vi "PH_SHS_Analysis.PC Global On.vi"(0 "i ref in":refnum<vi>, 2 "Global On?":bool, 5 "error in (no error)":errorcluster) -> (14 "i ref out":refnum<vi>, 19 "error out":errorcluster)   [LabVIEW 2014, in "PH_SHS_Analysis.lvlib"]
doc: "This is the Proc Case \"Remote Control\"."
uses:
  PH_SHS_Analysis.lvlib
  PH_Common/PH_Common.lvlib
  CSCore/BaseProcess/BaseProcess.lvlib
  PH_Img_BaseClass/PH_Img_BaseClass.lvlib
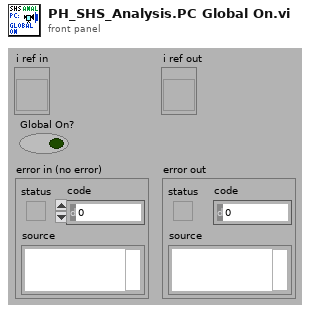
[diagram p1: front panel]
types:
  T1 = typedef "PH_SHS_Analysis.lvlib/PH_SHS_Analysis.i attribute.ctl" = cluster{"GUI Refs":cluster{"Delete":refnum<vi>, "Global On":refnum<vi>, "Cam Source":refnum<vi>, "Calibration Data File":refnum<vi>, "Calibration status":refnum<vi>, "Show overlay":refnum<vi>, "SHS Device Config":refnum<vi>, "Result":refnum<vi>, "Consider Tilt":refnum<vi>, "Working Reference":refnum<vi>, "Remove Tilt":refnum<vi>, "Take Cali  Reference":refnum<vi>, "Publishing Data Status":refnum<vi>, "Calibration Data":refnum<vi>}, "Calibration":cluster{"Status":T2, "Data":T3, "File":path}, "Result":T8, "Image":T11, "SHS Device Config":T12, "Show Overlay":bool, "GradientZernikeMatrix":dbl[][], "Consider Tilt":bool, "Working Reference":T4, "Zernicke Service ID":i32, "PSDB Image":T11}
  T2 = typedef "PH_StatusHandler.lvlib/PH_StatusHandler.Status.ctl" = i16
  T3 = typedef "PH_SHS_Analysis_Calibrator.lvlib/PH_SHS_Analysis_Calibrator.Analysis Calibration Data.ctl" = cluster{"Date":string, "Time":string, "Cam Settings":cluster{"Cam ID":string, "Gain":dbl, "Brightness":dbl, "Shutter":dbl, "Cam Error":bool, "Mode":i32}, "SHS Reference Result":T4, "Pixel Size":dbl, "MLA Pitch":dbl, "Method":enum16{"automatic", "manual"}, "Calibration Data calculated":bool, "No Problems at calculation?":bool, "error out":errorcluster}
  T4 = typedef "SHS_Common.lvlib/SHSReference.ctl" = cluster{"Reference":T5[][], "Lens Array Pitch [px]":dbl}
  T5 = typedef "SHS_Common.lvlib/ReferencePoint.ctl" = cluster{"Rect":T6, "Point":T7}
  T6 = typedef "SHS_Common.lvlib/Rectangle.ctl" = cluster{"Left":i32, "Top":i32, "Right":i32, "Bottom":i32}
  T7 = typedef "SHS_Common.lvlib/Point.ctl" = cluster{"x":dbl, "y":dbl, "valid?":bool, "weight":dbl}
  T8 = typedef "PH_SHS_Analysis.lvlib/PH_SHS_Analysis.Result.ctl" = cluster{"Time Stamp":timestamp, "Zernike Coefficients":T9, "PtV [lambda]":dbl, "Shifts":T10, "Measurement Quality":cluster{dbl, dbl, dbl}, "Measurement valid?":bool}
  T9 = typedef "PH_SHS_Analysis.lvlib/PH_SHS_Analysis.Zernike Coefficients.ctl" = cluster{"Tilt x":dbl, "Tilt y":dbl, "Defocus":dbl, "Astig 0°":dbl, "Astig 45°":dbl, "Coma x":dbl, "Coma y":dbl, "Spherical":dbl, "Trefoil 0°":dbl, "Trefoil 30°":dbl, "2nd Astig 0°":dbl, "2nd Astig 45°":dbl, "2nd Coma x":dbl, "2nd Coma y":dbl, "2nd Spherical":dbl}
  T10 = typedef "SHS_Common.lvlib/Shifts.ctl" = T7[][]
  T11 = typedef "IMAQ Image.ctl" = refnum<image>
  T12 = typedef "SHS_Analysis.lvlib/SHS_DeviceConfig.ctl" = cluster{"focal length [m]":dbl, "pixel size [m/px]":dbl, "wavelength [m]":dbl}
  T13 = typedef "PH_Img_BaseClass.lvlib/PH_Img_BaseClass.i attribute.ctl" = cluster{"GUI Refs":T14, "Timeout Image [ms]":i32, "Default Periodic Period [ms]":i32, "Camera":cluster{"Instancename":string, "Notifier":refnum<notifier>}, "Palette":T15, "Cam Settings":cluster{"Cam ID":string, "Gain":dbl, "Brightness":dbl, "Shutter":dbl, "Cam Info Failure":bool, "Mode":i32}}
  T14 = typedef "PH_Img_BaseClass.lvlib/PH_Img_BaseClass.GUI Refs.ctl" = cluster{"Timeout":refnum<vi>, "Image":refnum<vi>, "Palette":refnum<vi>, "Timeout Set":refnum<vi>}
  T15 = typedef "PH_Img_BaseClass.lvlib/PH_Img_BaseClass.Palette.ctl" = i32
  T16 = enum8{"Enabled", "Disabled", "Disabled and Grayed Out"}
  T17 = enum16{"simple", "synchronous", "asynchronous", "notification"}
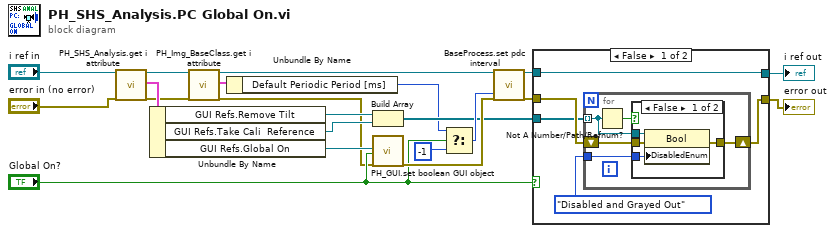
[diagram p0: block diagram]
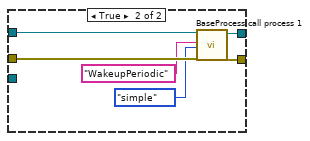
[diagram p3: hidden frame]
diagram:
  n1 = call "PH_SHS_Analysis.get i attribute.vi"("i ref in"="i ref in", "error in (no error)"="error in (no error)") -> ("i ref out"=w17:refnum<vi>, "i attribute"=w19:T1, "error out"=w4:errorcluster)  [unwired: 15 in]
  n2 = Unbundle By Name(w19) -> ("GUI Refs.Remove Tilt"=w8:refnum<vi>, "GUI Refs.Take Cali  Reference"=w7:refnum<vi>, "GUI Refs.Global On"=w18:refnum<vi>)
  n3 = call "PH_Img_BaseClass.get i attribute.vi"("i ref in"=w17, "error in (no error)"=w4) -> ("i ref out"=w5:refnum<vi>, "i attribute"=w2:T13, "error out"=w3:errorcluster)  [unwired: 15 in]
  n4 = Unbundle By Name(w2) -> ("Default Periodic Period [ms]"=w1:i32)
  n5 = Build Array(w8, w7) -> (w6:refnum<vi>[])
  n6 = call "PH_GUI.set boolean GUI object.vi"("Boolean Knob GUI Ref"=w18, "Value"="Global On?", "error in (no error)"=w3) -> ("error out"=w16:errorcluster)  [unwired: 16 in]
  n7 = Select(t=w1, s="Global On?", f=-1) -> (s? t:f=w14:i32)
  n8 = call "BaseProcess.set pdc interval.vi"("i ref in"=w5, "PeriodicInterval [ms]"=w14, "error in (no error)"=w16) -> ("i ref out"=w13:refnum<vi>, "error out"=w11:errorcluster)  [unwired: 14 in, 1 out]
  n9 = case shown="False" "Global On?" {
    tunnel: [w26 w42] -> w12
    tunnel: w11 -> [w24 w41]
    tunnel: [w23 w40] -> w10
    tunnel: w13 -> [w26 w39]
    tunnel: w6 -> [w22 _]
    frame False {
      n10 = for {
        tunnel: T16."Disabled and Grayed Out" ("Disabled") -> [w30]
        shift-right: [w28] -> w23
        shift-left: w24 -> [w29]
        tunnel: w22 -> [w27] mode=indexing
        n11 = Not A Number/Path/Refnum?(number/path/refnum=w27) -> (NaN/Path/Refnum?=w31:bool)
        n12 = case shown="False" w31 {
          tunnel: w29 -> [w35 w36]
          tunnel: [w34 w36] -> w28
          tunnel: w27 -> [w33 _]
          tunnel: w30 -> [w32 _]
          frame False {
            n13 = property class="Bool"(reference=w33, error in=w35, "DisabledEnum"=w32) -> (error out=w34:errorcluster)  [unwired: 1 out]
          }
          frame True {
          }
        }
      }
    }
    frame True {
      n14 = call "BaseProcess.call process 1.vi"("i ref in"=w39, "Selector"="WakeupPeriodic", "CallType"=T17."simple", "error in (no error)"=w41) -> ("i ref out"=w42:refnum<vi>, "error out"=w40:errorcluster)  [unwired: 13 in, 1 out]
    }
  }
  "i ref out" <- w12
  "error out" <- w10
